vi "GetVersion.vi"(8 "error in (no error)":errorcluster) -> (0 "error out":errorcluster)   [LabVIEW 2015, in "LabBassMOD2.lvlib"]
uses:
  LabBassMOD2.lvlib
  DLL/BASSMOD.dll
panel:
  out "return type":i32
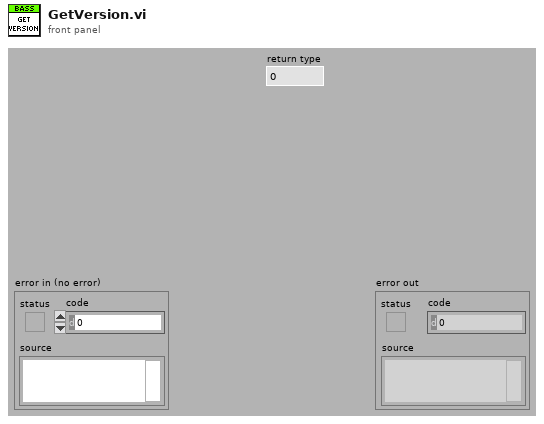
[diagram p1: front panel]
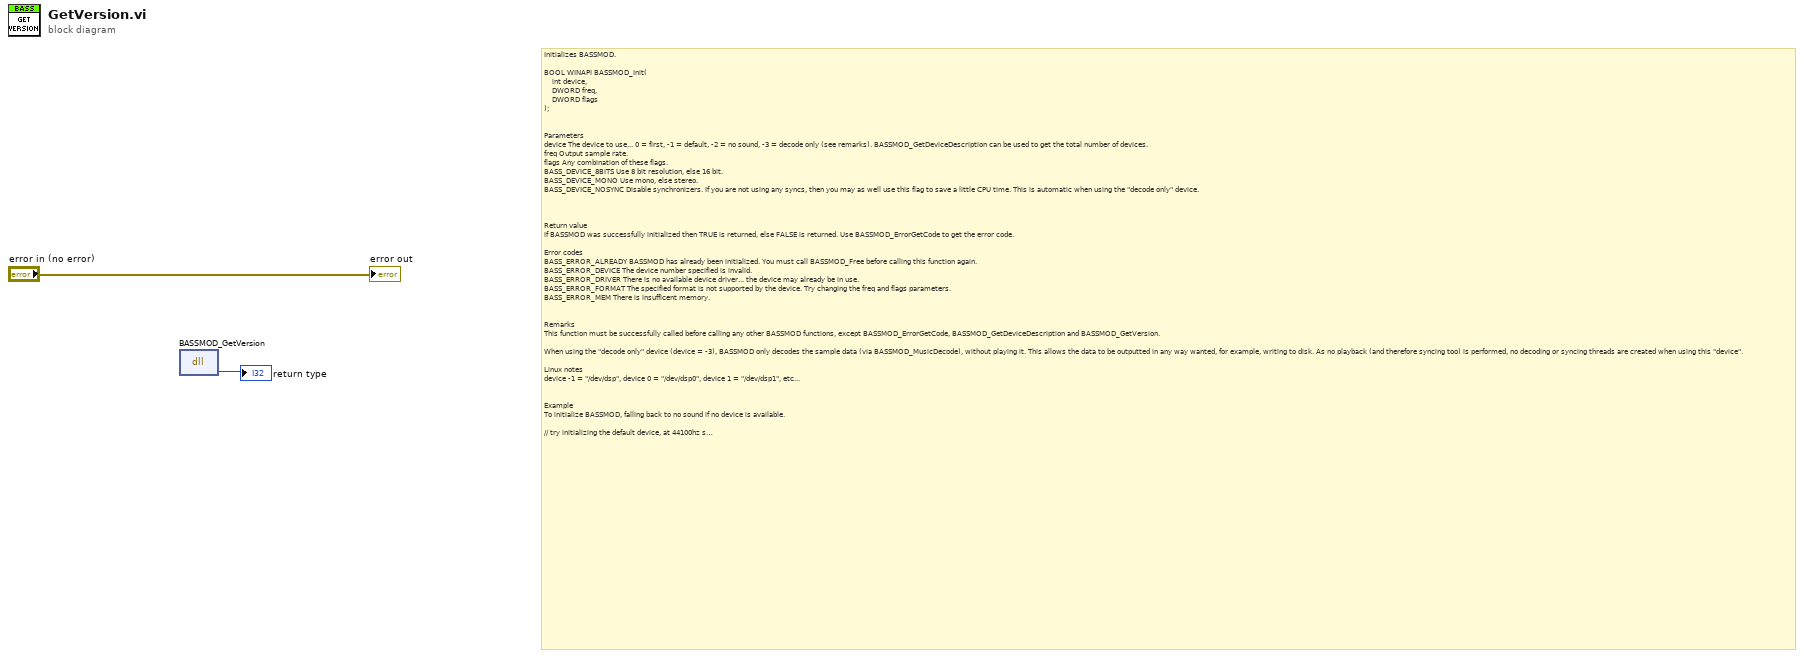
[diagram p0: block diagram]
diagram:
  # "Initializes BASSMOD.\n\nBOOL WINAPI BASSMOD_Init(\n    int device,\n    DWORD freq,\n    DWORD flags\n); \n\n\nParameters\ndevice The device to use... 0 = first, -1 = default, -2 = no sound, -3 = decode only (see remarks). BASSMOD_GetDeviceDescription can be used to get the total number of devices. \nfreq Output sample rate. \nflags Any combination of these flags.\nBASS_DEVICE_8BITS Use 8 bit resolution, else 16 bit.  \nBASS_DEVICE_MONO Use mono, else stereo.  \nBASS_DEVICE_NOSYNC Disable synchronizers. If you are not using any syncs, then you may as well use this flag to save a little CPU time. This is automatic when using the \"decode only\" device.  \n \n\n\nReturn value\nIf BASSMOD was successfully initialized then TRUE is returned, else FALSE is returned. Use BASSMOD_ErrorGetCode to get the error code.\n\nError codes\nBASS_ERROR_ALREADY BASSMOD has already been initialized. You must call BASSMOD_Free before calling this function again. \nBASS_ERROR_DEVICE The device number specified is invalid. \nBASS_ERROR_DRIVER There is no available device driver... the device may already be in use. \nBASS_ERROR_FORMAT The specified format is not supported by the device. Try changing the freq and flags parameters. \nBASS_ERROR_MEM There is insufficent memory. \n\n\nRemarks\nThis function must be successfully called before calling any other BASSMOD functions, except BASSMOD_ErrorGetCode, BASSMOD_GetDeviceDescription and BASSMOD_GetVersion.\n\nWhen using the \"decode only\" device (device = -3), BASSMOD only decodes the sample data (via BASSMOD_MusicDecode), without playing it. This allows the data to be outputted in any way wanted, for example, writing to disk. As no playback (and therefore syncing too) is performed, no decoding or syncing threads are created when using this \"device\".\n\nLinux notes\ndevice -1 = \"/dev/dsp\", device 0 = \"/dev/dsp0\", device 1 = \"/dev/dsp1\", etc... \n\n\nExample\nTo initialize BASSMOD, falling back to no sound if no device is available.\n\n// try initializing the default device, at 44100hz stereo 16 bits\nif (!BASSMOD_Init(-1,44100,0)) {\n    // couldn't initialize device, so use no sound\n    BASSMOD_Init(-2,44100,0)\n} \n\n\nSee also\nBASSMOD_Free, BASSMOD_MusicLoad, BASSMOD_SetVolume"
  n1 = dll-call lib="C:/dev/PGS/LabBASSMOD2/DLL/BASSMOD.dll" fn="BASSMOD_GetVersion"() -> ("return type"=→"return type":i32)  [unwired: 3 in, 2 out]
  "error out" <- "error in (no error)"
